vi "midi_ParseEvent.vi"(9 "input cluster":T1={"status"=0, "channel"=0, "data byte 1"=0, "data byte 2"=0, "tempo"=500000, "track name"="0", "text"=""}, 11 "string":string) -> (1 "output cluster":T1={"status"=15, "channel"=15, "data byte 1"=0, "data byte 2"=0, "tempo"=0, "track name"="", "text"=""}, 3 "result string":string)   [LabVIEW 2013]
panel:
  out "s? t:f":string
  # "midi_ParseEvent"
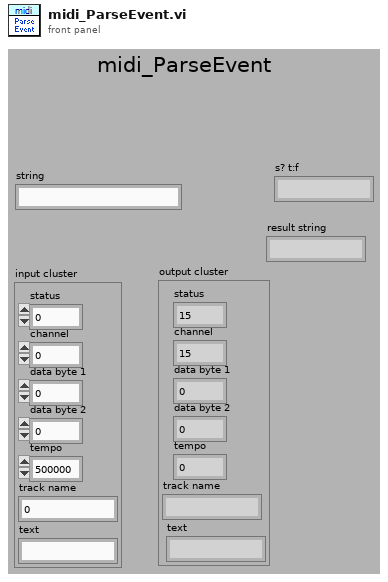
[diagram p1: front panel]
types:
  T1 = cluster{"status":u8, "channel":u8, "data byte 1":u8, "data byte 2":u8, "tempo":u32, "track name":string, "text":string}
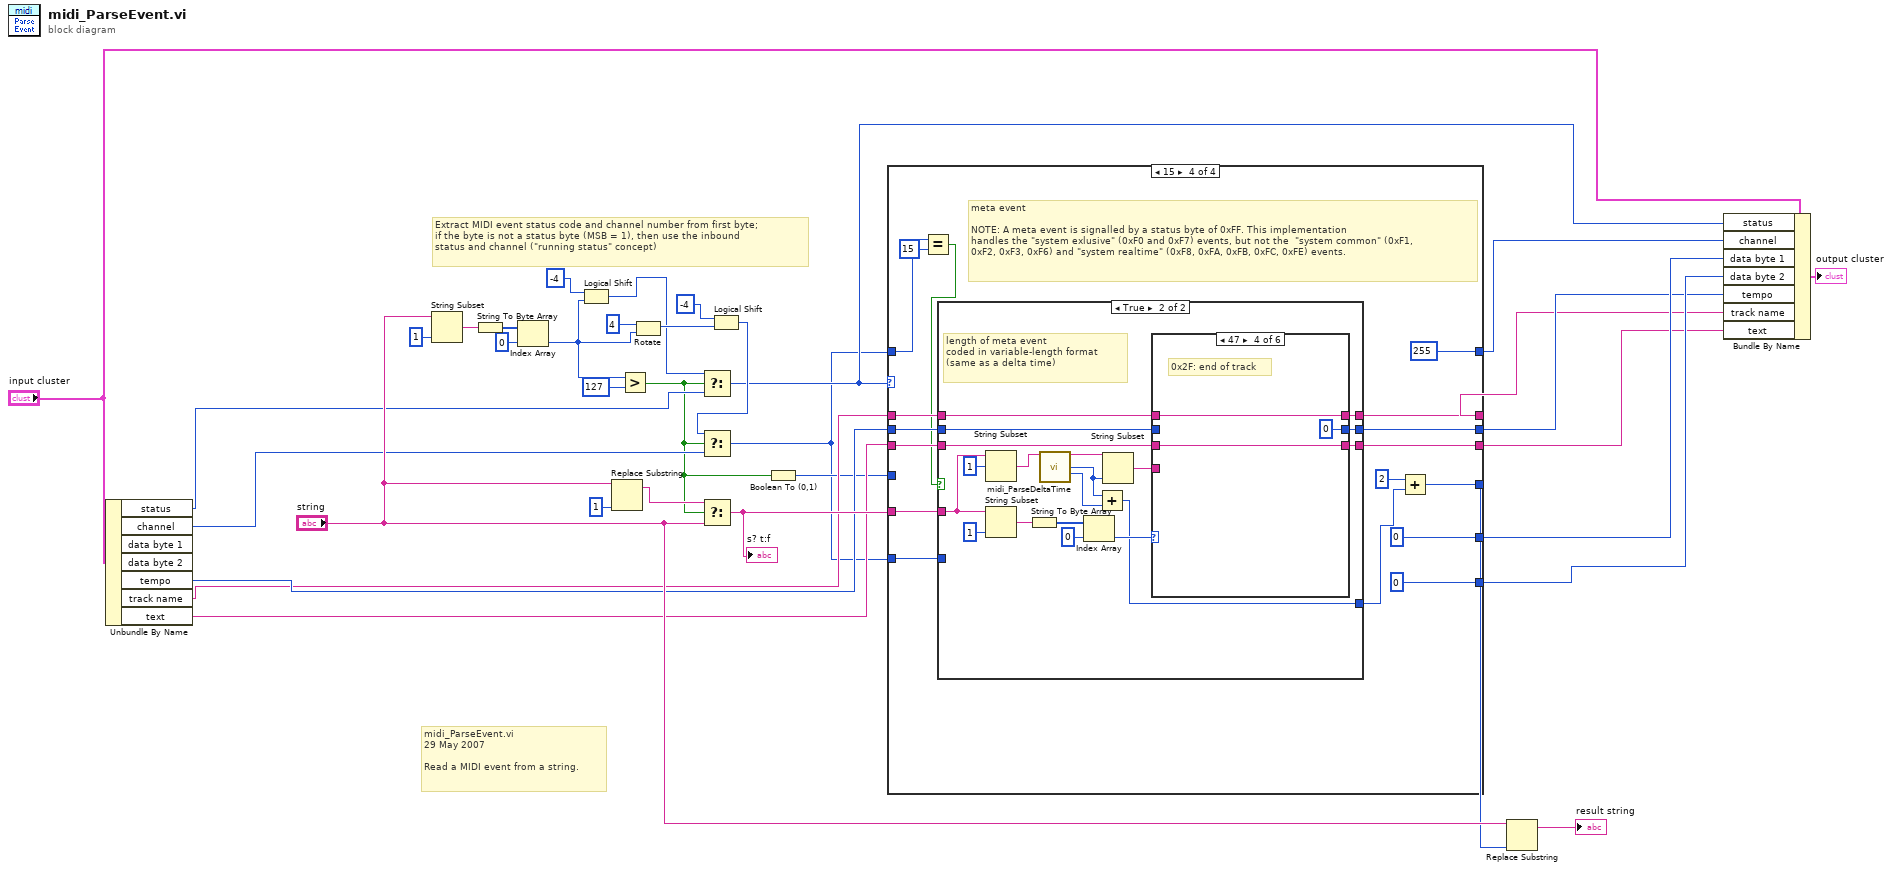
[diagram p0: block diagram]
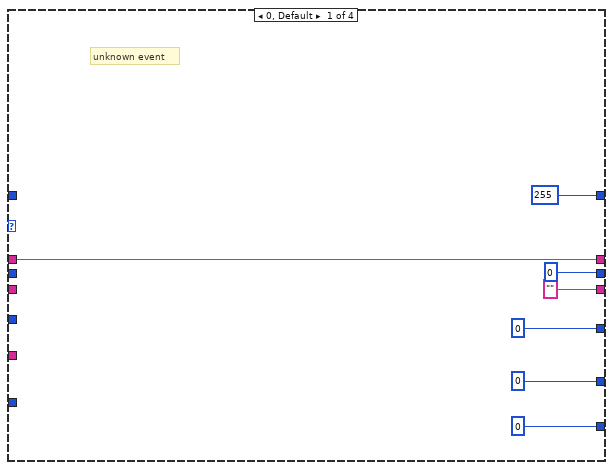
[diagram p2: hidden frame]
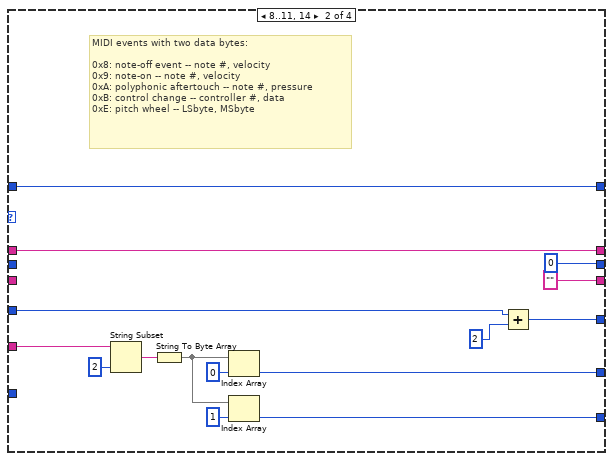
[diagram p3: hidden frame]
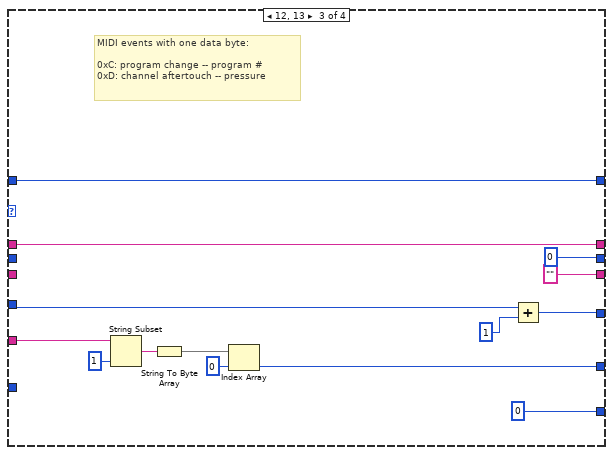
[diagram p4: hidden frame]
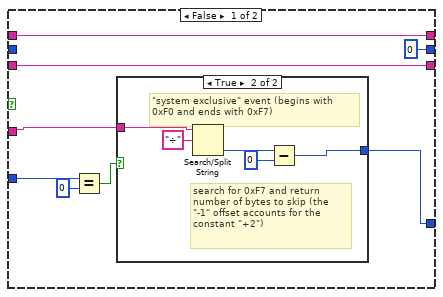
[diagram p5: hidden frame]
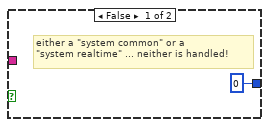
[diagram p6: hidden frame]
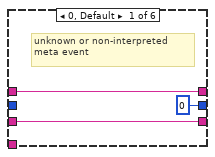
[diagram p7: hidden frame]
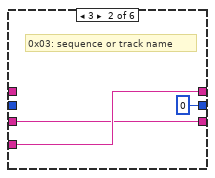
[diagram p8: hidden frame]
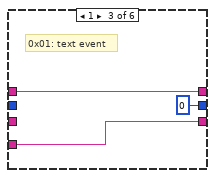
[diagram p9: hidden frame]
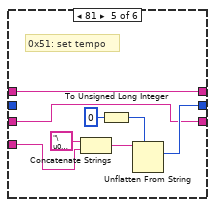
[diagram p10: hidden frame]
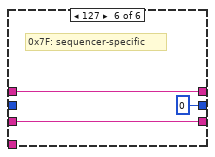
[diagram p11: hidden frame]
diagram:
  # "Extract MIDI event status code and channel number from first byte;\nif the byte is not a status byte (MSB = 1), then use the inbound\nstatus and channel (\"running status\" concept)"
  # "midi_ParseEvent.vi\n29 May 2007\n\nRead a MIDI event from a string."
  n1 = Unbundle By Name("input cluster") -> ("status"=w11:u8, "channel"=w9:u8, "tempo"=w8:u32, "track name"=w7:string, "text"=w5:string)  [unwired: 2 out]
  n2 = String Subset(string="string", length (rest)=1 ("length (rest)")) -> (substring=w33:string)  [unwired: 1 in]
  n3 = String To Byte Array(string=w33) -> (unsigned byte array=w32:u8[])
  n4 = Index Array(array=w32, index=0) -> (element=w27:u8)
  n5 = Logical Shift(y=-4 ("length (rest)"), x=w27) -> (x << y=w25:u8)
  n6 = Replace Substring(2:1 ("length (len. of substring)"), 5:"string") -> (1:w22:string)  [unwired: 2 in, 1 out]
  n7 = Greater?(x=w27, y=u8 127) -> (0:w3:bool)
  n8 = Rotate(1:w27, 2:i16 4 ("y")) -> (0:w28:u8)
  n9 = Select(t=w25, s=w3, f=w11) -> (s? t:f=w17:u8)
  n10 = Select(t=w22, s=w3, f="string") -> (s? t:f=w21:string)
  "s? t:f" <- w21
  n11 = Logical Shift(y=-4 ("length (rest)"), x=w28) -> (x << y=w24:u8)
  n12 = Select(t=w24, s=w3, f=w9) -> (s? t:f=w2:u8)
  n13 = Boolean To (0,1)(Boolean=w3) -> (0, 1=w4:i16)
  n14 = case shown="15" w17 {
    tunnel: w21 -> [_ w54 w68 w87]
    tunnel: [u8 0 w51 w66 u8 0] -> w16
    tunnel: [u8 0 w50 u8 0 u8 0] -> w15
    tunnel: [0 ("index") w46 w62 w82] -> w19
    tunnel: w8 -> [_ _ _ w86]
    tunnel: [u32 0 u32 0 u32 0 w85] -> w14
    tunnel: [w39 w49 w64 w80] -> w13
    tunnel: w7 -> [w39 w49 w64 w79]
    tunnel: w4 -> [_ w47 w61 _]
    tunnel: ["" ("text") "" ("text") "" ("text") w78] -> w6
    tunnel: w5 -> [_ _ _ w77]
    tunnel: w2 -> [_ w44 w59 w76]
    tunnel: w2 -> [_ _ _ w73]
    tunnel: [u8 255 ("channel") w44 w59 u8 255 ("channel")] -> w1
    frame 0, Default {
      # "unknown event"
    }
    frame 8..11, 14 {
      # "MIDI events with two data bytes:\n\n0x8: note-off event -- note #, velocity\n0x9: note-on -- note #, velocity\n0xA: polyphonic aftertouch -- note #, pressure\n0xB: control change -- controller #, data\n0xE: pitch wheel -- LSbyte, MSbyte"
      n15 = String Subset(string=w54, length (rest)=2 ("length (rest)")) -> (substring=w56:string)  [unwired: 1 in]
      n16 = String To Byte Array(string=w56) -> (unsigned byte array=w52:u8[])
      n17 = Index Array(array=w52, index=0) -> (element=w51:u8)
      n18 = Index Array(array=w52, index=1) -> (element=w50:u8)
      n19 = Add(x=w47, y=2 ("index")) -> (x+y=w46:i32)
    }
    frame 12, 13 {
      # "MIDI events with one data byte:\n\n0xC: program change -- program # \n0xD: channel aftertouch -- pressure"
      n20 = String Subset(string=w68, length (rest)=1 ("length (rest)")) -> (substring=w70:string)  [unwired: 1 in]
      n21 = String To Byte Array(string=w70) -> (unsigned byte array=w67:u8[])
      n22 = Index Array(array=w67, index=0) -> (element=w66:u8)
      n23 = Add(x=w61, y=1 ("index")) -> (x+y=w62:i32)
    }
    frame 15 {
      # "meta event\n\nNOTE: A meta event is signalled by a status byte of 0xFF. This implementation\nhandles the \"system exlusive\" (0xF0 and 0xF7) events, but not the  \"system common\" (0xF1,\n0xF2, 0xF3, 0xF6) and \"system realtime\" (0xF8, 0xFA, 0xFB, 0xFC, 0xFE) events."
      n24 = Equal?(x=w76, y=u8 15) -> (x = y?=w74:bool)
      n25 = case shown="True" w74 {
        tunnel: w87 -> [w94 w114]
        tunnel: w86 -> [_ w112]
        tunnel: [u32 0 w111] -> w85
        tunnel: [w90 w107] -> w81
        tunnel: [w96 w106] -> w80
        tunnel: w79 -> [w96 w105]
        tunnel: [w95 w104] -> w78
        tunnel: w77 -> [w95 w103]
        tunnel: w73 -> [w92 _]
        frame False {
          n26 = Equal?(x=w92, y=u8 0) -> (x = y?=w91:bool)
          n27 = case shown="True" w91 {
            tunnel: w94 -> [_ w101]
            tunnel: [0 ("offset of match") w100] -> w90
            frame False {
              # "either a \"system common\" or a \n\"system realtime\" ... neither is handled!"
            }
            frame True {
              # "search for 0xF7 and return\nnumber of bytes to skip (the\n\"-1\" offset accounts for the\nconstant \"+2\")"
              # "\"system exclusive\" event (begins with\n0xF0 and ends with 0xF7)"
              n28 = Search/Split String(string=w101, search string/char (-)="÷") -> (offset of match=w99:i32)  [unwired: 1 in, 2 out]
              n29 = Subtract(x=w99, y=0) -> (x-y=w100:i32)
            }
          }
        }
        frame True {
          # "length of meta event\ncoded in variable-length format\n(same as a delta time)"
          n30 = String Subset(string=w114, offset (0)=1) -> (substring=w116:string)  [unwired: 1 in]
          n31 = String Subset(string=w114, length (rest)=1 ("length (rest)")) -> (substring=w119:string)  [unwired: 1 in]
          n32 = String To Byte Array(string=w119) -> (unsigned byte array=w121:u8[])
          n33 = call "midi_ParseDeltaTime.vi"("string"=w116) -> ("result string"=w113:string, "delta time (tics)"=w109:u32, "bytes read"=w108:i32)  [unwired: 11 in, 1 out]
          n34 = Index Array(array=w121, index=0) -> (element=w115:u8)
          n35 = Add(x=w109, y=w108) -> (x+y=w107:u32)
          n36 = String Subset(string=w113, length (rest)=w109) -> (substring=w110:string)  [unwired: 1 in]
          n37 = case shown="47" w115 {
            tunnel: w112 -> [_ _ _ _ _ _]
            tunnel: [u32 0 u32 0 u32 0 u32 0 w139 u32 0] -> w111
            tunnel: w110 -> [_ w127 w129 _ w137 _]
            tunnel: [w124 w127 w130 w133 w135 w144] -> w106
            tunnel: w105 -> [w124 _ w130 w133 w135 w144]
            tunnel: [w123 w126 w129 w132 w134 w143] -> w104
            tunnel: w103 -> [w123 w126 _ w132 w134 w143]
            frame 0, Default {
              # "unknown or non-interpreted\nmeta event"
            }
            frame 3 {
              # "0x03: sequence or track name"
            }
            frame 1 {
              # "0x01: text event"
            }
            frame 47 {
              # "0x2F: end of track"
            }
            frame 81 {
              # "0x51: set tempo"
              n38 = Concatenate Strings("\u0000" ("string"), w137) -> (w136:string)
              n39 = To Unsigned Long Integer(number=u32 0) -> (unsigned 32bit integer=w140:u32)
              n40 = Unflatten From String(type=w140, binary string=w136) -> (value=w139:u32)  [unwired: 3 in, 2 out]
            }
            frame 127 {
              # "0x7F: sequencer-specific"
            }
          }
        }
      }
      n41 = Add(x=u32 2, y=w81) -> (x+y=w82:u32)
    }
  }
  n42 = Replace Substring(2:w19, 5:"string") -> (1:→"result string":string)  [unwired: 2 in, 1 out]
  n43 = Bundle By Name(cluster="input cluster", "status"=w17, "channel"=w1, "data byte 1"=w16, "data byte 2"=w15, "tempo"=w14, "track name"=w13, "text"=w6) -> (→"output cluster":T1)
